vi "Colorimetro.vi"() -> ()   [LabVIEW 2013]
uses:
  <vilib>/Instr/_visa.llb/Select Event Type.ctl
  <vilib>/Analysis/3filter.llb/Savitzky-Golay Filter (DBL).vi
  <vilib>/Instr/_visa.llb/VISA Configure Serial Port (Instr).vi
  <vilib>/Analysis/NI_AALBase.lvlib
  <vilib>/Analysis/NI_AALPro.lvlib
panel:
  in  "Colore":u8(ring) items=["GREEN", "RED", "BLUE"]
  out "Punto min ms":dbl
  out "Punto MAX ms":dbl
  in  "Tab Control":enum32{"Colore", "Derivata Filtrata"}(tab)
  out "XY Graph":cluster{i32[], i32[]}(graph)
  out "XY Graph 2":cluster{i32[], "Filtered X":dbl[]}(graph)
  in  "stop":bool
  out "Luce B":dbl
  out "Luce G":dbl
  out "Luce R":dbl
  out "Luce nf":dbl
  out "Tempo ms":dbl
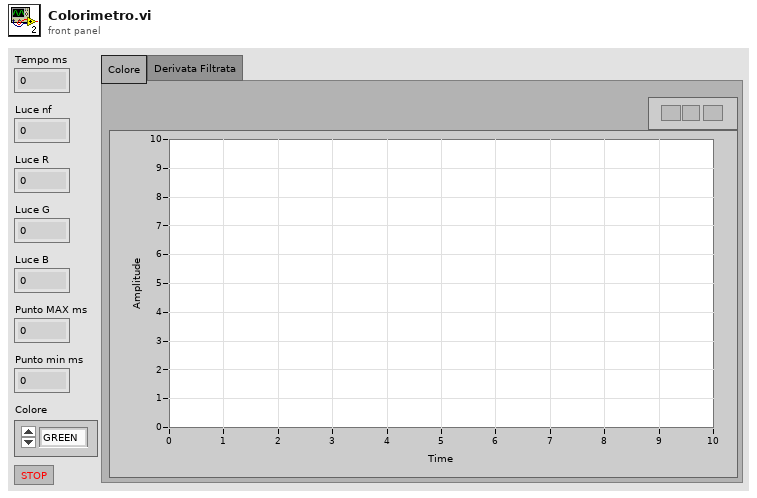
[diagram p1: front panel]
types:
  T1 = typedef "Select Event Type.ctl" = u32
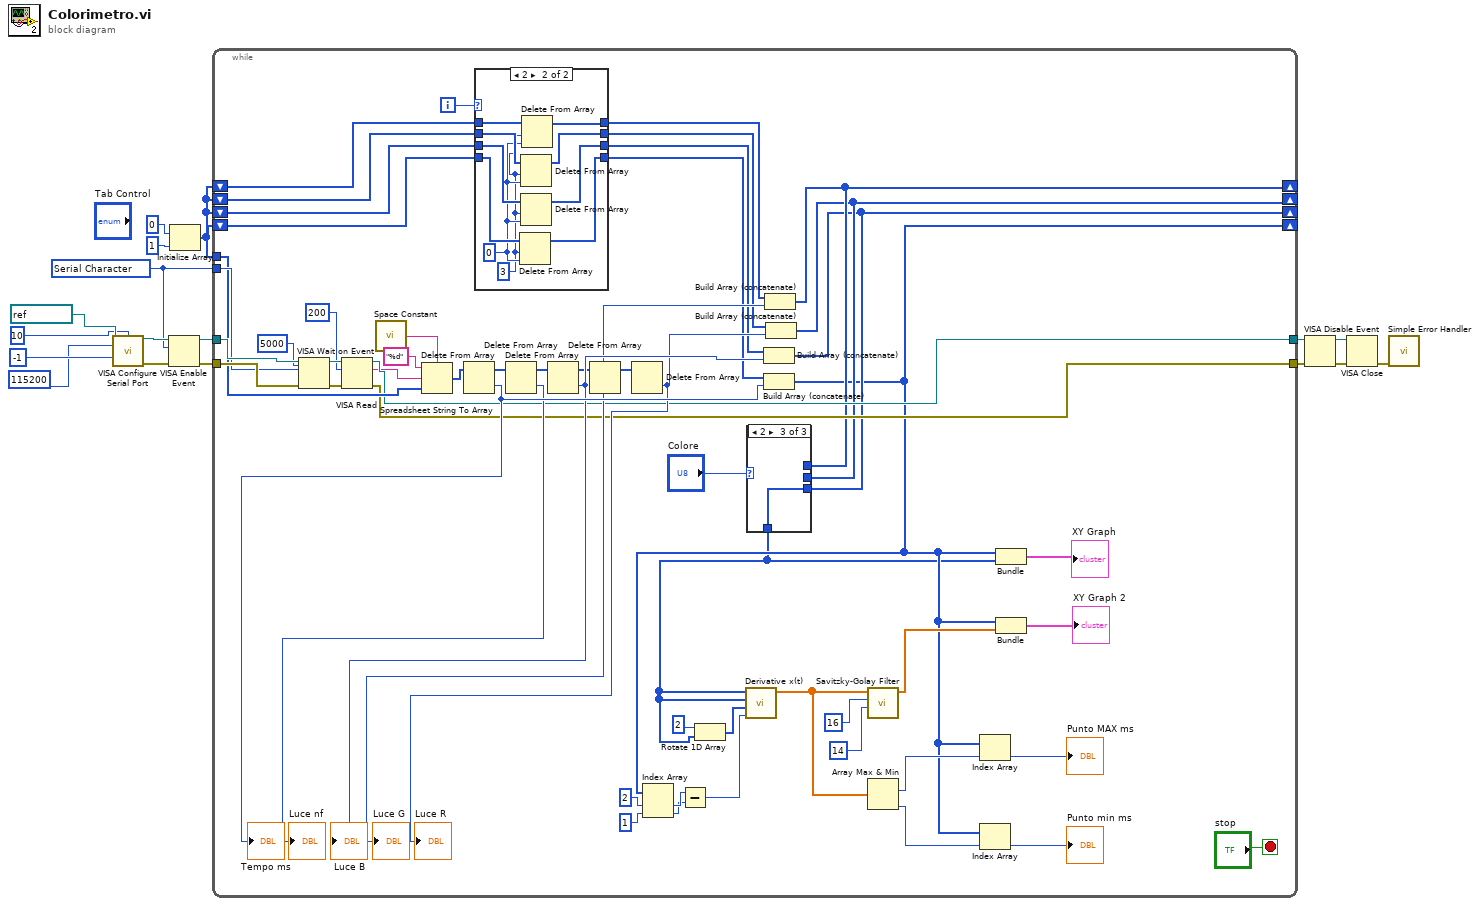
[diagram p0: block diagram]
diagram:
  w12 = T1 1073684533 items=["Service Request"=1073684491, "Trigger"=3221168138, "Clear"=1073684493, "VXI Signal"=1073684512, "VXI/VME Interrupt"=3221168161, "VXI/VME Sysfail"=1073684509, "VXI/VME Sysreset"=1073684510, "GPIB CIC"=1073684498, "GPIB Talk"=1073684499, "GPIB Listen"=1073684500, "PXI Interrupt"=1073684514, "Serial Break"=1073684515, "Serial TermChar"=1073684516, "Serial CTS"=1073684521, "Serial DSR"=1073684522, "Serial DCD"=1073684524, "Serial RI"=1073684526, "Serial Character"=1073684533, "USB Interrupt"=1073684535, "All Enabled"=1073709055] ("Event Type")
  n1 = call-poly "VISA Configure Serial Port"("VISA resource name"=refnum<visa-resource-name> "COM5", "timeout (10sec)"=-1, "termination char\n(0xA = '\\n' = LF)"=10, "baud rate (9600)"=115200) -> ("VISA resource name out"=w16:refnum<visa-resource-name>, "error out"=w15:errorcluster)  [unwired: 10 in]
  n2 = VISA Enable Event(8:w15, 10:w12, 11:w16) -> (0:w13:errorcluster, 3:w14:refnum<visa-resource-name>)  [unwired: 1 in]
  n3 = Initialize Array(0, 1) -> (w9:i32[])
  n4 = while {
    tunnel: w14 -> [w73]
    tunnel: w13 -> [w72]
    tunnel: w12 -> [w71]
    tunnel: w9 -> [w65]
    shift-right: [w35] -> _
    shift-left: w9 -> [w27]
    shift-right: [w36] -> _
    shift-left: w9 -> [w29]
    shift-right: [w38] -> _
    shift-left: w9 -> [w33]
    shift-right: [w37] -> _
    shift-left: w9 -> [w31]
    tunnel: [w55] -> w5
    tunnel: [w54] -> w4
    i -> [w34]
    stop <- "stop" stop-if-true
    n5 = VISA Wait on Event(7:5000, 8:w72, 10:w71, 11:w73) -> (0:w69:errorcluster, 3:w68:refnum<visa-resource-name>)  [unwired: 1 in, 2 out]
    n6 = VISA Read(VISA resource name=w68, byte count=200, error in (no error)=w69) -> (VISA resource name out=w55:refnum<visa-resource-name>, read buffer=w53:string, error out=w54:errorcluster)  [unwired: 1 out]
    n7 = call <vilib>:"Space Constant.vi"() -> ("String"=w50:string)
    n8 = Spreadsheet String To Array(delimiter (Tab)=w50, format string="%d", spreadsheet string=w53, array type (2D Dbl)=w65) -> (array=w52:i32[])
    n9 = Delete From Array(array=w52) -> (deleted portion=w64:i32, array with subset deleted=w51:i32[])  [unwired: 2 in]
    "Tempo ms" <- w64
    n10 = case shown="2" w34 {
      tunnel: w33 -> [w77 w84]
      tunnel: w31 -> [w76 w85]
      tunnel: w29 -> [w75 w86]
      tunnel: w27 -> [w74 w87]
      tunnel: [w77 w83] -> w32
      tunnel: [w76 w82] -> w30
      tunnel: [w75 w81] -> w28
      tunnel: [w74 w80] -> w26
      frame 0, Default {
      }
      frame 2 {
        w78 = 3
        w79 = 0
        n11 = Delete From Array(array=w87, length=w78, index=w79) -> (array with subset deleted=w80:i32[])  [unwired: 1 out]
        n12 = Delete From Array(array=w85, length=w78, index=w79) -> (array with subset deleted=w82:i32[])  [unwired: 1 out]
        n13 = Delete From Array(array=w86, length=w78, index=w79) -> (array with subset deleted=w81:i32[])  [unwired: 1 out]
        n14 = Delete From Array(array=w84, length=w78, index=w79) -> (array with subset deleted=w83:i32[])  [unwired: 1 out]
      }
    }
    n15 = Delete From Array(array=w51) -> (deleted portion=→"Luce nf":i32, array with subset deleted=w62:i32[])  [unwired: 2 in]
    n16 = Delete From Array(array=w62) -> (deleted portion=w61:i32, array with subset deleted=w60:i32[])  [unwired: 2 in]
    "Luce B" <- w61
    n17 = Delete From Array(array=w60) -> (deleted portion=w59:i32, array with subset deleted=w58:i32[])  [unwired: 2 in]
    "Luce G" <- w59
    n18 = Delete From Array(array=w58) -> (deleted portion=w57:i32)  [unwired: 2 in, 1 out]
    "Luce R" <- w57
    n19 = Build Array (concatenate)(w28, w61) -> (w36:i32[])
    n20 = Build Array (concatenate)(w26, w64) -> (w35:i32[])
    n21 = Index Array(array=w35, index #1=2, index #2=1) -> (element #1=w46:i32, element #2=w45:i32)
    n22 = Subtract(x=w46, y=w45) -> (x-y=w44:i32)
    n23 = Build Array (concatenate)(w32, w59) -> (w38:i32[])
    n24 = Build Array (concatenate)(w30, w57) -> (w37:i32[])
    n25 = case shown="2" "Colore" {
      tunnel: w38 -> [w88 w89 _]
      tunnel: [w88 w89 w90] -> w18
      tunnel: w37 -> [_ _ _]
      tunnel: w36 -> [_ _ w90]
      frame 0, Default {
      }
      frame 1 {
      }
      frame 2 {
      }
    }
    n26 = Rotate 1D Array(1:w18, 2:2) -> (0:w19:i32[])
    n27 = call <vilib>:"Derivative x(t).vi"("dt"=w44, "Final Condition"=w19, "Initial Condition"=w18, "X"=w18) -> ("dX/dt"=w43:dbl[])  [unwired: 1 in, 6 out]
    n28 = call-poly <vilib>:"Savitzky-Golay Filter.vi"("polynomial order"=14, "side points"=16, "X"=w43) -> ("Filtered X"=w49:dbl[])  [unwired: 1 in, 7 out]
    n29 = Array Max & Min(array=w43) -> (max index (indices)=w42:i32, min index (indices)=w41:i32)  [unwired: 2 out]
    n30 = Index Array(array=w35, index=w42) -> (element=→"Punto MAX ms":i32)
    n31 = Index Array(array=w35, index=w41) -> (element=→"Punto min ms":i32)
    n32 = Bundle(w35, w18) -> (→"XY Graph":cluster{i32[], i32[]})  [unwired: 1 in]
    n33 = Bundle(w35, "Filtered X"=w49) -> (→"XY Graph 2":cluster{i32[], "Filtered X":dbl[]})  [unwired: 1 in]
  }
  n34 = VISA Disable Event(8:w4, 11:w5) -> (0:w8:errorcluster, 3:w7:refnum<visa-resource-name>)  [unwired: 1 in, 1 out]
  n35 = VISA Close(VISA resource name=w7, error in (no error)=w8) -> (error out=w6:errorcluster)
  n36 = call <vilib>:"Simple Error Handler.vi"("error in (no error)"=w6) -> ()  [unwired: 1 in, 8 out]
